vi "RT_AIChar_v2.vi"() -> ()   [LabVIEW 2019]
uses:
  FPGA/TypeDefs/SamplingModeEnum.ctl
  FPGA/TypeDefs/AO mode TabCtrl.ctl
  <vilib>/NI/STM/SubVIs/MetaDataElement.ctl
  <vilib>/Platform/TimedLoop/XDataNode/timing_clust.ctl
  <vilib>/Platform/TimedLoop/XDataNode/nitl_modes.ctl
  <vilib>/Platform/TimedLoop/XDataNode/wakeup.ctl
  <vilib>/rvi/Analysis/host/Butterworth/config/Butterworth Filter Order.ctl
  <vilib>/rvi/Analysis/host/Butterworth/config/Butterworth Filter Type.ctl
  <vilib>/NI/STM/TCP/Write Meta Data (TCP Ref).vi
  <vilib>/NI/STM/TCP/Get Connection Reference (TCP).vi
  <vilib>/NI/STM/TCP/Write Meta Data (TCP Clst).vi
  <vilib>/FPGAPlugInAG/myRIO-1900/niLvFpga_Open_myRIO-1900.vi
  <vilib>/rvi/interface/common/dynamic/niFpgaDynamicAddResources.vi
  <vilib>/NI/STM/TCP/Write Message (TCP).vi
  <vilib>/rvi/Analysis/host/Private/Sample Rate To Loop Time (ticks).vi
  <vilib>/rvi/Analysis/host/Butterworth/config/BwScaledCoefficients.vi
  <vilib>/Utility/error.llb/Error Cluster From Error Code.vi
  <vilib>/rvi/errors/niLvFpgaAdjustHostInterfaceError.vi
  <vilib>/FPGAPlugInAG/Dynamic/niLvFpga_Close_Dynamic.vi
  <vilib>/rvi/interface/nirviOpenFPGA/nirviOpenFPGA.xnode
  FPGA Bitfiles/adc,dacnoisemeas_FPGATarget_FPGAMainv3_mK2rDMr4N+c.lvbitx
  <vilib>/rvi/Analysis/host/Butterworth/XNode/ButterworthCoefficients.xnode
  <vilib>/rvi/interface/nirviReadWriteControl/nirviReadWriteControl.xnode
  <vilib>/Platform/TimedLoop/XDataNode/XDataNode.xnode
  <vilib>/rvi/interface/nirviCloseFPGA/nirviCloseFPGA.xnode
  <vilib>/Platform/TimedLoop/XDataNode/XDNodeRunTimeDep.lvlib
  Components/Timing/Timing.lvlib
  <vilib>/NI/STM/NI STM.lvlib
  NiFpgaLv.dll
  <vilib>/rvi/interface/Simulation/niFpgaSimulationCallBeginRW.vi
  <vilib>/rvi/Analysis/host/Public/NI_FpgaMspHost.lvlib
panel:
  in  "AO mode":T1=enum."100*AI"
  in  "AO Out [V]":fxp<+/-,18,5>
  in  "AI-chain LPF [Hz]":dbl=1000.0 format="%#_6p"
  in  "Sampling Mode":T2
  out "Sample Time\ntoo small?":bool
  in  "AO enable?":bool
  in  "Sample Freq [Hz]":dbl=333000.0 format="%#.3p"
  out "RT Loop Rate":dbl format="%.3p"
  out "# of iterations\n[STM write]":i32
  out "# elements \nFIFO buffer":u32
  out "Finished \nlate counter?":dbl
  in  "stop":bool
  # "- Open PC_SensorChar vi and run that VI as well to start capturing data!\n- Sampling Mode : \n     - LPF adds a  butterworth filter after the ADC conversion.\n     - 4pt. Avg adds a 4pt. Moving Avg before the LPF and after ADC."
  # "AO = \n100 * (AI value)"
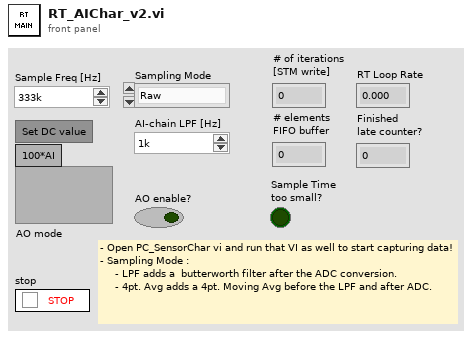
[diagram p1: front panel]
types:
  T1 = typedef "AO mode TabCtrl.ctl" = enum32{"Set DC value", "100*AI"}
  T2 = typedef "SamplingModeEnum.ctl" = enum16{"Raw", "LPF", "4 pt. Avg. + LPF"}
  T3 = typedef "NI STM.lvlib/MetaDataElement.ctl" = string
  T4 = typedef "NI STM.lvlib/TCP Connection Info.ctl" = cluster{"connection ID":refnum<k5>, "meta data":T3[]}
  T5 = typedef "XDNodeRunTimeDep.lvlib/timing_clust.ctl" = cluster{"Expected End [f-1]":u64, "Actual End [f-1]":u64, "Finished Late? [f-1]":bool, "Expected End [i-1]":u64, "Actual End [i-1]":u64, "Finished Late? [i-1]":bool, "Expected Start [i]":u64, "Actual Start [i]":u64, "Expected Start [f]":u64, "Actual Start [f]":u64, "Source Name":string, "Structure Name":string, "Period":i64, "Deadline":i64, "Offset":i64, "Start":i64, "Priority":i32, "Timeout":i32, "Mode":T6, "Wakeup Reason":T7, "Error":errorcluster, "Source Type":string, "Secondary Source Type":string, "Global End Time":u64, "Global Start Time":u64, "Frame Duration":u64, "Iteration Duration":u64, "Assigned CPU":i32, "I/O Scan Engine Mode":u32}
  T6 = typedef "XDNodeRunTimeDep.lvlib/nitl_modes.ctl" = enum32{"No Change", "Process missed periods, maintain original phase", "Discard missed periods, maintain original phase", "Process missed periods, ignore original phase", "Discard missed periods, ignore original phase"}
  T7 = typedef "XDNodeRunTimeDep.lvlib/wakeup.ctl" = enum32{"Normal", "Aborted", "Asynchronous wakeup", "Timing source error", "Timed loop error", "Timeout"}
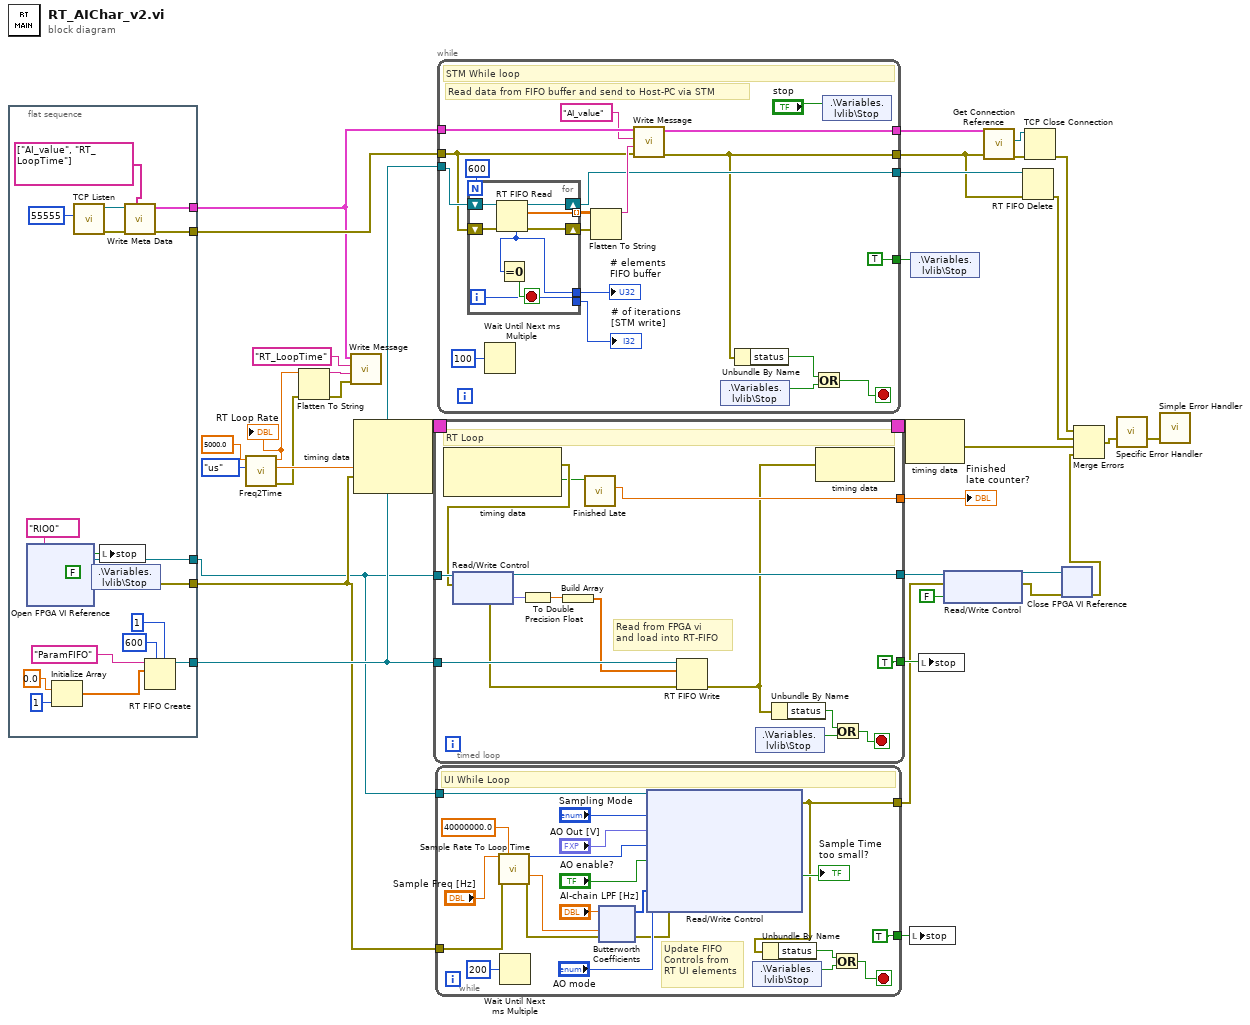
[diagram p0: block diagram]
diagram:
  n1 = flat-sequence {
    tunnel: [w51] -> w8
    tunnel: [w50] -> w7
    tunnel: [w45] -> w21
    tunnel: [w44] -> w29
    tunnel: [w43] -> w25
    frame #0 {
      w52 = FALSE ("Stop")
      n2 = xnode "Open FPGA VI Reference"("resource name"=tag "RIO0") -> ("FPGA VI Reference Out"=w50:refnum<k20>, "error out"=w53:errorcluster)  [unwired: 1 in]
      n3 = Initialize Array(0.0 ("element"), 1 ("dimension size")) -> (w38:dbl[])
      n4 = call <vilib>:"TCP Listen.vi"("port"=u16 55555) -> ("error out"=w48:errorcluster, "connection ID"=w47:refnum<k5>)  [unwired: 6 in, 3 out]
      n5 = shared-variable ".\\Variables.lvlib\\Stop"(w52, error in=w53) -> (error out=w51:errorcluster)
      n6 = local write "stop"(w52) -> ()
      n7 = call-poly <vilib>:"Write Meta Data.vi"("meta data"=T3[] ["AI_value", "RT_LoopTime"], "error in"=w48, "connection ID"=w47) -> ("error out"=w44:errorcluster, "connection info out"=w45:T4)  [unwired: 7 in]
      n8 = RT FIFO Create(0:"ParamFIFO" ("name (unnamed)"), 1:w38, 4:u32 600 ("size (10)"), 6:u32 1 ("elements in array (1)")) -> (8:w43:refnum<k33>)  [unwired: 4 in, 2 out]
    }
  }
  n9 = call "Freq2Time.vi"("Int. Time Unit"=enum16{"sec", "us", "ms"}."us", "Sample rate (Hz)"=5000.0 ("Period")) -> ("error out"=w15:errorcluster, "Int.  time [unit]"=w30:dbl, "New Sample rate (Hz)"=w17:dbl)  [unwired: 7 in]
  "RT Loop Rate" <- w17
  n10 = Flatten To String(anything=w17, error in (no error)=w15) -> (data string=w18:string, error out=w19:errorcluster)  [unwired: 2 in, 1 out]
  n11 = call-poly <vilib>:"Write Message.vi"("error in"=w19, "data"=w18, "name"="RT_LoopTime", "connection info in"=w21) -> ()  [unwired: 6 in, 2 out]
  n12 = node-c288(w30, w8) -> (w35:T5)  [unwired: 1 in]
  n13 = timed-loop {
    tunnel: w7 -> [w68]
    timing: w35 -> [_]
    timing-out: [_] -> w34
    tunnel: [w65] -> w33
    tunnel: w25 -> [w64]
    tunnel: [TRUE ("Stop")] -> w5
    tunnel: [w58] -> w6
    stop <- w57 stop-if-true
    # "Read from FPGA vi \nand load into RT-FIFO"
    # "RT Loop"
    n14 = node-c288() -> (w67:errorcluster, w66:bool)  [unwired: 1 in]
    n15 = xnode "Read/Write Control"("FPGA VI Reference In"=w68, "error in"=w67) -> ("FPGA VI Reference Out"=w58:refnum<k20>, "error out"=w59:errorcluster, "AI In [V]"=w63:fxp<+/-,25,5>)
    n16 = To Double Precision Float(number=w63) -> (double precision float=w62:dbl)
    n17 = Build Array(w62) -> (w61:dbl[])
    n18 = call "Finished Late.vi"("Finished \nLate?"=w66) -> ("# Finished\nLate counter"=w65:dbl)  [unwired: 8 in, 2 out]
    n19 = RT FIFO Write(0:w64, 1:w61, 3:w59) -> (11:w54:errorcluster)  [unwired: 2 in, 3 out]
    n20 = shared-variable ".\\Variables.lvlib\\Stop"() -> (w56:bool)  [unwired: 1 in, 1 out]
    n21 = Unbundle By Name(w54) -> ("status"=w55:bool)
    n22 = node-c288(w54) -> ()  [unwired: 1 out]
    n23 = Or(x=w55, y=w56) -> (x .or. y?=w57:bool)
  }
  "Finished \nlate counter?" <- w33
  n24 = while {
    tunnel: w8 -> [w81]
    tunnel: w7 -> [w89]
    tunnel: [TRUE ("Stop")] -> w4
    tunnel: [w76] -> w3
    stop <- w78 stop-if-true
    # "Update FIFO \nControls from\nRT UI elements"
    # "UI While Loop"
    n25 = call-poly <vilib>:"Sample Rate To Loop Time.vi"("sample rate (S/s)"="Sample Freq [Hz]", "FPGA clock rate (Hz)"=40000000.0, "error in (no error)"=w81) -> ("count (ticks/S)"=w83:u32, "actual sample rate (S/s)"=w82:dbl, "error out"=w80:errorcluster)  [unwired: 10 in]
    n26 = Wait Until Next ms Multiple(millisecond multiple=u32 200) -> ()  [unwired: 1 out]
    n27 = xnode "Butterworth Coefficients"("cutoff frequency (Hz)"="AI-chain LPF [Hz]", "sample rate (S/s)"=w82, "error in (no error)"=w80) -> ("scaled coefficients"=w93:i32[], "error out"=w75:errorcluster)
    n28 = xnode "Read/Write Control"("FPGA VI Reference In"=w89, "error in"=w75, "Sampling Mode"="Sampling Mode", "AO Out [V]"="AO Out [V]", "Sample Time [ticks]"=w83, "AO enable?"="AO enable?", "Scaled Butterworth Coeffs"=w93, "AO mode"="AO mode") -> ("error out"=w76:errorcluster, "FPGA AO DMA Overflow?"=→"Sample Time\ntoo small?":bool)  [unwired: 1 out]
    n29 = shared-variable ".\\Variables.lvlib\\Stop"() -> (w79:bool)  [unwired: 1 in, 1 out]
    n30 = Unbundle By Name(w76) -> ("status"=w77:bool)
    n31 = Or(x=w77, y=w79) -> (x .or. y?=w78:bool)
  }
  n32 = while {
    tunnel: w21 -> [w120]
    tunnel: w29 -> [w113]
    tunnel: [w118] -> w28
    tunnel: [w103] -> w23
    tunnel: w25 -> [w115]
    tunnel: [w112] -> w24
    tunnel: [TRUE ("Stop")] -> w1
    stop <- w105 stop-if-true
    # "Read data from FIFO buffer and send to Host-PC via STM"
    # "STM While loop"
    n33 = for {
      N: 600 -> [_]
      shift-right: [w126] -> w112
      shift-left: w115 -> [w129]
      shift-right: [w128] -> w114
      shift-left: w113 -> [w127]
      tunnel: [w125] -> w111
      tunnel: [w123] -> w110
      tunnel: [w122] -> w109 mode=indexing
      i -> [w123]
      stop <- w124 stop-if-true
      n34 = RT FIFO Read(0:w129, 3:w127) -> (7:w125:u32, 8:w126:refnum<k33>, 9:w122:dbl[], 11:w128:errorcluster)  [unwired: 2 in, 1 out]
      n35 = Equal To 0?(x=w125) -> (x = 0?=w124:bool)
    }
    "# elements \nFIFO buffer" <- w111
    "# of iterations\n[STM write]" <- w110
    n36 = Wait Until Next ms Multiple(millisecond multiple=u32 100) -> ()  [unwired: 1 out]
    n37 = Flatten To String(anything=w109, error in (no error)=w114) -> (data string=w117:string)  [unwired: 2 in, 2 out]
    n38 = call-poly <vilib>:"Write Message.vi"("error in"=w113, "data"=w117, "name"="AI_value", "connection info in"=w120) -> ("error out"=w103:errorcluster, "connection info out"=w118:T4)  [unwired: 6 in]
    n39 = shared-variable ".\\Variables.lvlib\\Stop"() -> (w106:bool)  [unwired: 1 in, 1 out]
    n40 = Unbundle By Name(w103) -> ("status"=w104:bool)
    n41 = Or(x=w104, y=w106) -> (x .or. y?=w105:bool)
    n42 = shared-variable ".\\Variables.lvlib\\Stop"("stop") -> ()  [unwired: 1 in, 1 out]
  }
  n43 = node-c288(w34) -> (w16:errorcluster)
  n44 = local write "stop"(w4) -> ()
  n45 = shared-variable ".\\Variables.lvlib\\Stop"(w1) -> ()  [unwired: 1 in, 1 out]
  n46 = local write "stop"(w5) -> ()
  n47 = xnode "Read/Write Control"("FPGA VI Reference In"=w6, "error in"=w3, "AO enable?"=FALSE ("AO enabled?")) -> ("FPGA VI Reference Out"=w11:refnum<k20>, "error out"=w10:errorcluster)
  n48 = call-poly <vilib>:"Get Connection Reference.vi"("error in"=w23, "connection info in"=w28) -> ("error out"=w27:errorcluster, "connection ID out"=w26:refnum<k5>)  [unwired: 7 in, 1 out]
  n49 = RT FIFO Delete(0:w24, 3:w23) -> (11:w22:errorcluster)  [unwired: 1 in]
  n50 = TCP Close Connection(connection ID=w26, error in (no error)=w27) -> (error out=w12:errorcluster)  [unwired: 1 in, 1 out]
  n51 = xnode "Close FPGA VI Reference"("FPGA VI Reference In"=w11, "error in"=w10) -> ("error out"=w2:errorcluster)
  n52 = Merge Errors(w12, w22, w16, w2) -> (w14:errorcluster)
  n53 = call "Specific Error Handler"("Error to Check"=w14) -> ("error out"=w13:errorcluster)  [unwired: 11 in, 3 out]
  n54 = call <vilib>:"Simple Error Handler.vi"("error in (no error)"=w13) -> ()  [unwired: 4 in, 5 out]
